vi "munormalizada.vi"(4 "Array":u32[][](array[numeric])) -> (14 "un02":dbl, 18 "un03":dbl, 19 "un30":dbl, 21 "un11":dbl, 23 "un12":dbl, 25 "un20":dbl, 27 "un21":dbl)   [LabVIEW 2021]
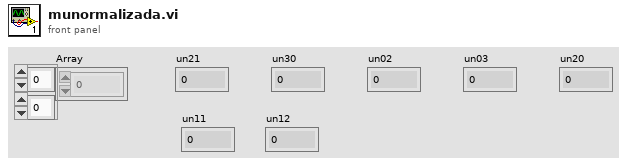
[diagram p1: front panel]
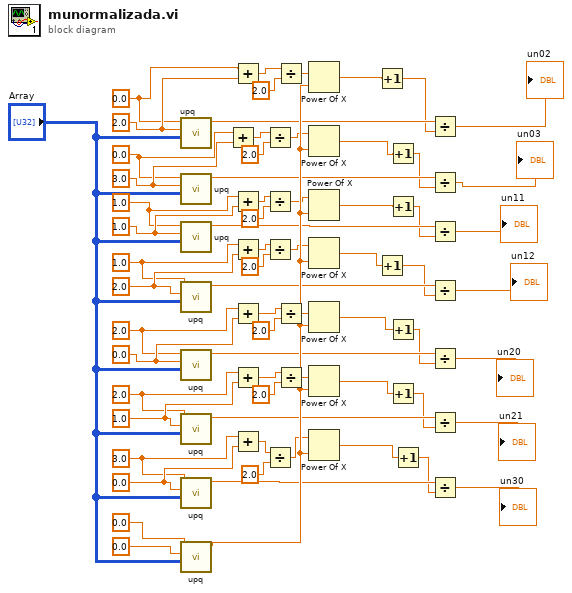
[diagram p0: block diagram]
diagram:
  w47 = 2.0 ("q")
  w46 = 0.0 ("p")
  w49 = 3.0 ("q")
  w48 = 0.0 ("p")
  w51 = 1.0 ("q")
  w50 = 1.0 ("p")
  w59 = 0.0 ("q")
  w58 = 3.0 ("p")
  w57 = 1.0 ("q")
  w56 = 2.0 ("p")
  w55 = 0.0 ("q")
  w54 = 2.0 ("p")
  w53 = 2.0 ("q")
  w52 = 1.0 ("p")
  n1 = call "upq.vi"("ImagenBinaria"="Array", "q"=w47, "p"=w46) -> ("upq"=w32:dbl)  [unwired: 8 in]
  n2 = call "upq.vi"("ImagenBinaria"="Array", "q"=w49, "p"=w48) -> ("upq"=w33:dbl)  [unwired: 8 in]
  n3 = call "upq.vi"("ImagenBinaria"="Array", "q"=w51, "p"=w50) -> ("upq"=w37:dbl)  [unwired: 8 in]
  n4 = call "upq.vi"("ImagenBinaria"="Array", "q"=w53, "p"=w52) -> ("upq"=w31:dbl)  [unwired: 8 in]
  n5 = call "upq.vi"("ImagenBinaria"="Array", "q"=w55, "p"=w54) -> ("upq"=w34:dbl)  [unwired: 8 in]
  n6 = call "upq.vi"("ImagenBinaria"="Array", "q"=w57, "p"=w56) -> ("upq"=w35:dbl)  [unwired: 8 in]
  n7 = call "upq.vi"("ImagenBinaria"="Array", "q"=w59, "p"=w58) -> ("upq"=w36:dbl)  [unwired: 8 in]
  n8 = call "upq.vi"("ImagenBinaria"="Array", "q"=0.0, "p"=0.0) -> ("upq"=w60:dbl)  [unwired: 8 in]
  n9 = Add(x=w48, y=w49) -> (x+y=w26:dbl)
  n10 = Add(x=w46, y=w47) -> (x+y=w28:dbl)
  n11 = Add(x=w50, y=w51) -> (x+y=w23:dbl)
  n12 = Add(x=w52, y=w53) -> (x+y=w22:dbl)
  n13 = Add(x=w54, y=w55) -> (x+y=w20:dbl)
  n14 = Add(x=w56, y=w57) -> (x+y=w18:dbl)
  n15 = Add(x=w58, y=w59) -> (x+y=w16:dbl)
  n16 = Divide(x=w26, y=2.0) -> (x/y=w25:dbl)
  n17 = Divide(x=w23, y=2.0) -> (x/y=w24:dbl)
  n18 = Divide(x=w22, y=2.0) -> (x/y=w21:dbl)
  n19 = Divide(x=w16, y=2.0) -> (x/y=w15:dbl)
  n20 = Divide(x=w28, y=2.0) -> (x/y=w27:dbl)
  n21 = Divide(x=w20, y=2.0) -> (x/y=w19:dbl)
  n22 = Divide(x=w18, y=2.0) -> (x/y=w17:dbl)
  n23 = Power Of X(1:w60, 2:w27) -> (0:w14:dbl)
  n24 = Power Of X(1:w60, 2:w25) -> (0:w9:dbl)
  n25 = Power Of X(1:w60, 2:w24) -> (0:w10:dbl)
  n26 = Power Of X(1:w60, 2:w21) -> (0:w4:dbl)
  n27 = Power Of X(1:w60, 2:w19) -> (0:w11:dbl)
  n28 = Power Of X(1:w60, 2:w17) -> (0:w12:dbl)
  n29 = Power Of X(1:w60, 2:w15) -> (0:w2:dbl)
  n30 = Increment(x=w14) -> (x+1=w13:dbl)
  n31 = Increment(x=w4) -> (x+1=w3:dbl)
  n32 = Increment(x=w9) -> (x+1=w8:dbl)
  n33 = Increment(x=w10) -> (x+1=w7:dbl)
  n34 = Increment(x=w11) -> (x+1=w6:dbl)
  n35 = Increment(x=w12) -> (x+1=w5:dbl)
  n36 = Increment(x=w2) -> (x+1=w1:dbl)
  n37 = Divide(x=w32, y=w13) -> (x/y=→"un02":dbl)
  n38 = Divide(x=w33, y=w8) -> (x/y=→"un03":dbl)
  n39 = Divide(x=w37, y=w7) -> (x/y=→"un11":dbl)
  n40 = Divide(x=w31, y=w3) -> (x/y=→"un12":dbl)
  n41 = Divide(x=w34, y=w6) -> (x/y=→"un20":dbl)
  n42 = Divide(x=w35, y=w5) -> (x/y=→"un21":dbl)
  n43 = Divide(x=w36, y=w1) -> (x/y=→"un30":dbl)
